vi "_error.vi"(8 "error in (no error)":errorcluster, 10 "Additional message":string, 11 "Status":T1) -> (0 "error out":errorcluster)   [LabVIEW 2013, in "LVAutomationListener.lvlib" / "LVAutomationListener.lvclass"]
uses:
  LVAutomationListener.lvclass
  _status.ctl
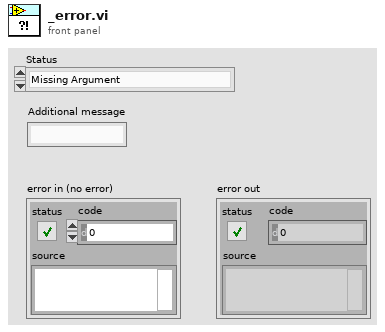
[diagram p1: front panel]
types:
  T1 = typedef "LVAutomationListener.lvlib/LVAutomationListener.lvclass/_status.ctl" = enum16{"Missing Argument", "Unknown Command", "Missing Build Spec Item", "Bad Type", "Compiler Aborted"}
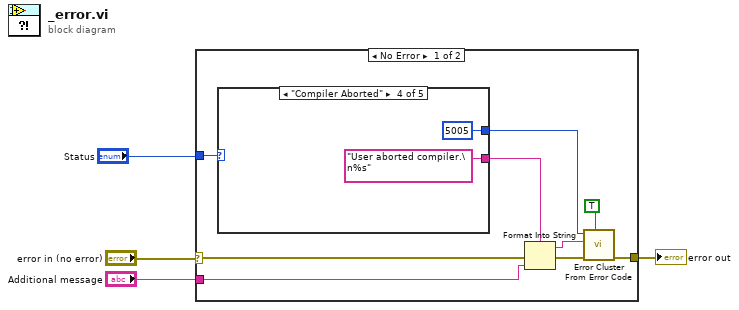
[diagram p0: block diagram]
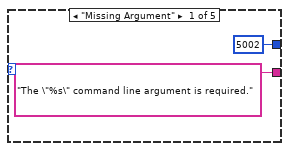
[diagram p2: hidden frame]
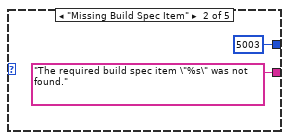
[diagram p3: hidden frame]
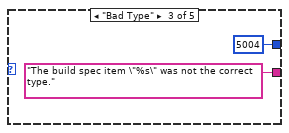
[diagram p4: hidden frame]
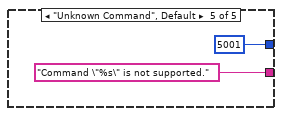
[diagram p5: hidden frame]
diagram:
  n1 = case shown="No Error" "error in (no error)" {
    selector: "error in (no error)" -> [w12 w24]
    tunnel: "Status" -> [w13 _]
    tunnel: "Additional message" -> [w10 _]
    tunnel: [w5 w24] -> w1
    frame No Error {
      n2 = case shown="\"Compiler Aborted\"" w13 {
        tunnel: ["The \"%s\" command line argument is required." "The required build spec item \"%s\" was not found." "The build spec item \"%s\" was not the correct type." "User aborted compiler.\n%s" "Command \"%s\" is not supported."] -> w11
        tunnel: [5002 5003 5004 5005 5001] -> w7
        frame "Missing Argument" {
        }
        frame "Missing Build Spec Item" {
        }
        frame "Bad Type" {
        }
        frame "Compiler Aborted" {
        }
        frame "Unknown Command", Default {
        }
      }
      n3 = Format Into String(format string=w11, error in=w12, w10) -> (resulting string=w8:string, error out=w9:errorcluster)  [unwired: 1 in]
      n4 = call <vilib>:"Error Cluster From Error Code.vi"("show call chain? (False)"=TRUE, "error in (no error)"=w9, "error message (\"\")"=w8, "error code (0)"=w7) -> ("error out"=w5:errorcluster)  [unwired: 5 in]
    }
    frame Error {
    }
  }
  "error out" <- w1
